vi "About Panther Dashboard.vi"(8 "error in":errorcluster) -> (0 "error out":errorcluster)   [LabVIEW 2019, in "Panther Dashboard.lvlib"]
uses:
  Panther Dashboard.lvlib
  <vilib>/Platform/browser.llb/Open URL in Default Browser (string).vi
panel:
  out "Title":string
  in  "Website":bool
  in  "About DQMH":bool
  out "DQMH Version:":string
  # "Developed and maintained by \nPantherLAB"
  # "Developer:\n\n» CLA & LabVIEW Champion                                           Enrique Noé Arias\n\nBrainstorming & Code Reviews (Alphabetical order):\n\n» Matthias Baudot\n» Fabiola De La Cueva\n» Christopher Farmer\n» Cyril Gambini\n» GDevCON NA\n» Joerg Hampel\n» Olivier Jourdan\n» Casey May\n» Cesar Muñoz\n» Darren Nattinger\n» Luis Orozco\n» Sam Taggart\n» Diego Torres"
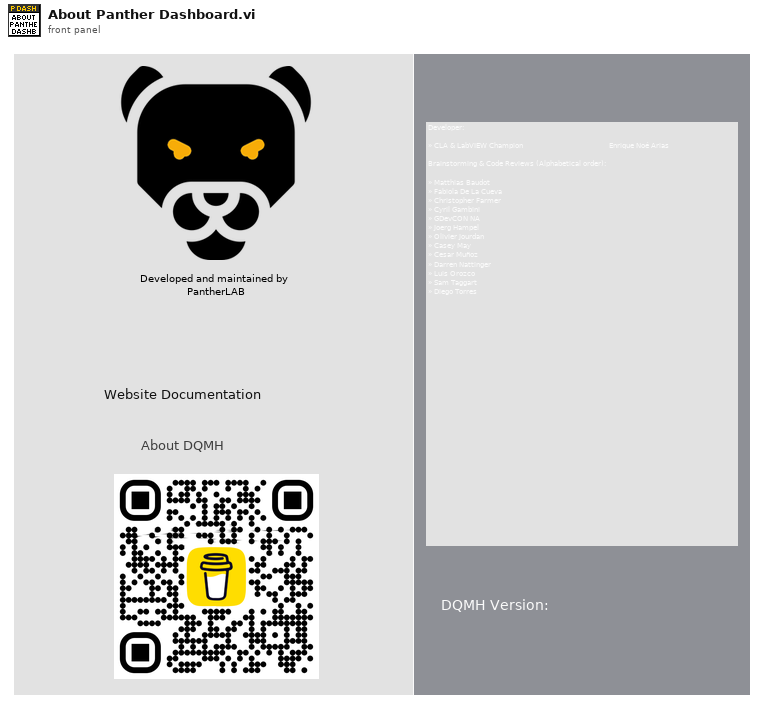
[diagram p1: front panel]
types:
  T1 = cluster{"Major":u16, "Minor":u16, "Fix":u16, "Build":u16}
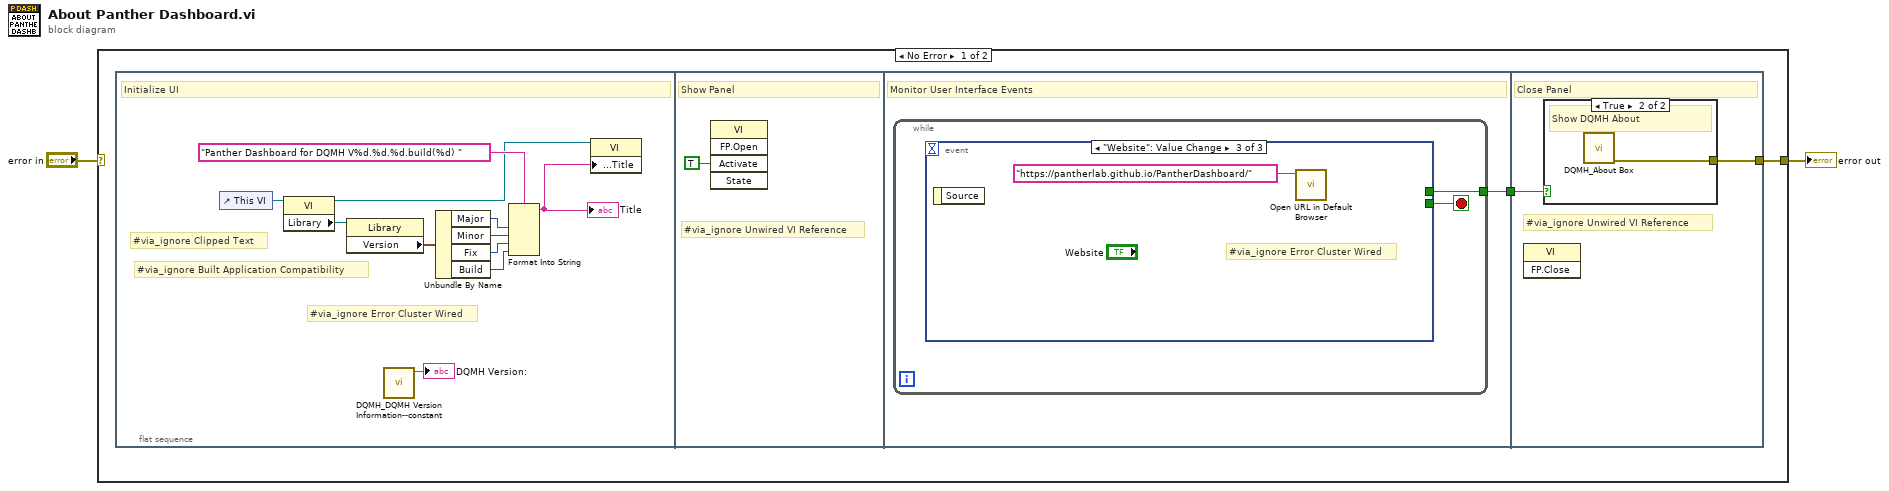
[diagram p0: block diagram]
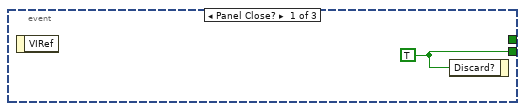
[diagram p2: hidden frame]
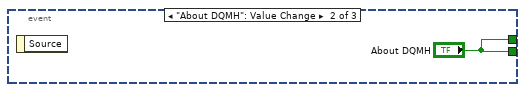
[diagram p3: hidden frame]
diagram:
  n1 = case shown="No Error" "error in" {
    selector: "error in" -> [_ w26]
    tunnel: [w4 w26] -> w1
    frame No Error {
      n2 = flat-sequence {
        tunnel: [w17] -> w3
        tunnel: w3 -> [w23]
        tunnel: [w24] -> w4
        frame #0 {
          # "#via_ignore Clipped Text"
          # "#via_ignore Built Application Compatibility"
          # "#via_ignore Error Cluster Wired"
          # "Initialize UI"
          n3 = control-ref of="This VI"() -> (w14:refnum<vi>)
          n4 = property class="VI"(reference=w14) -> (reference out=w7:refnum<vi>, "Library"=w13:refnum<vi>)  [unwired: 1 in, 1 out]
          n5 = property class="Library"(reference=w13) -> ("Version"=w12:T1)  [unwired: 1 in, 2 out]
          n6 = call <vilib>:"DQMH_DQMH Version Information--constant.vi"() -> ("DQMH Version"=→"DQMH Version:":string)  [unwired: 11 in]
          n7 = Unbundle By Name(w12) -> ("Major"=w11:u16, "Minor"=w10:u16, "Fix"=w9:u16, "Build"=w8:u16)
          n8 = Format Into String(format string="Panther Dashboard for DQMH V%d.%d.%d.build(%d) " ("String"), w11, w10, w9, w8) -> (resulting string=w6:string)  [unwired: 2 in, 1 out]
          "Title" <- w6
          n9 = property class="VI"(reference=w7, "Front Panel.Title"=w6) -> ()  [unwired: 1 in, 2 out]
        }
        frame #1 {
          # "#via_ignore Unwired VI Reference"
          # "Show Panel"
          n10 = invoke class="VI" method="FP.Open"("Activate"=TRUE ("Activate?")) -> ()  [unwired: 4 in, 5 out]
        }
        frame #2 {
          # "Monitor User Interface Events"
          n11 = while {
            tunnel: [w18] -> w17
            stop <- w19 stop-if-true
            n12 = event shown="[2] \"Website\": Value Change" {
              selector: _ -> [_ _ _]
              dyn-events: _ -> [_ _ _]
              timeout: _ -> [_ _ _]
              tunnel: [w20 "About DQMH" _] -> w19
              tunnel: [_ "About DQMH" _] -> w18
              event Panel Close? {
                w20 = TRUE ("Discard?")
                n13 = event-data() -> ()  [unwired: 1 in, 1 out]
                n14 = event-data("Discard?"=w20) -> ()  [unwired: 1 in, 1 out]
              }
              event "About DQMH": Value Change {
                n15 = event-data() -> ()  [unwired: 1 in, 1 out]
              }
              event "Website": Value Change {
                # "#via_ignore Error Cluster Wired"
                n16 = event-data() -> ()  [unwired: 1 in, 1 out]
                n17 = call-poly <vilib>:"Open URL in Default Browser.vi"("URL"="https://pantherlab.github.io/PantherDashboard/") -> ()  [unwired: 5 in, 2 out]
              }
            }
          }
        }
        frame #3 {
          # "#via_ignore Unwired VI Reference"
          # "Close Panel"
          n18 = invoke class="VI" method="FP.Close"() -> ()  [unwired: 3 in, 3 out]
          n19 = case shown="True" w23 {
            tunnel: [_ w25] -> w24
            frame False {
            }
            frame True {
              # "Show DQMH About"
              n20 = call <vilib>:"DQMH_About Box.vi"() -> ("error out"=w25:errorcluster)  [unwired: 11 in]
            }
          }
        }
      }
    }
    frame Error {
    }
  }
  "error out" <- w1
